vi "Color_Min_Max_ISOSPI.vi"(9 "datain":dbl[][](array[numeric]), 10 "valeur invalide":dbl, 11 "Table en entrée":refnum<vi>) -> ()   [LabVIEW 2020]
uses:
  <vilib>/Utility/miscctls.llb/LVRowAndColumnTypeDef.ctl
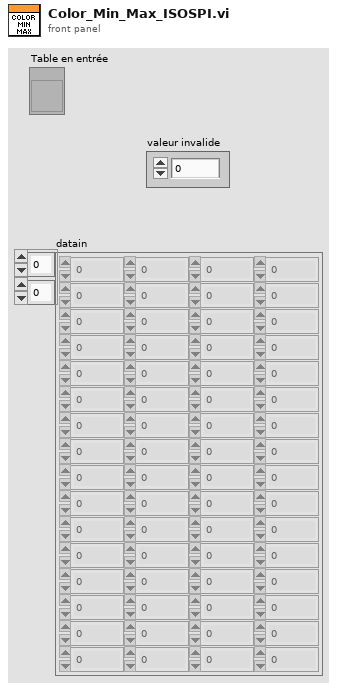
[diagram p1: front panel]
types:
  T1 = typedef "LVRowAndColumnTypeDef.ctl" = cluster{"Row":i32, "Column":i32}
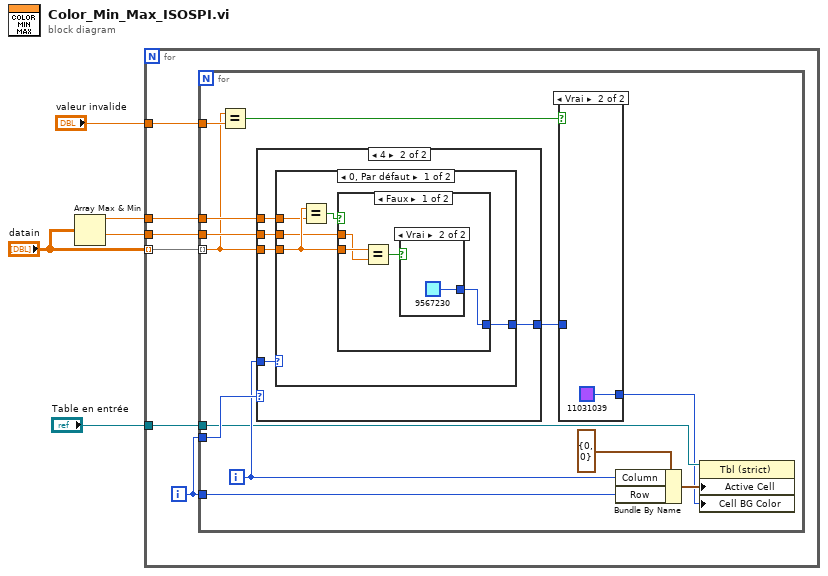
[diagram p0: block diagram]
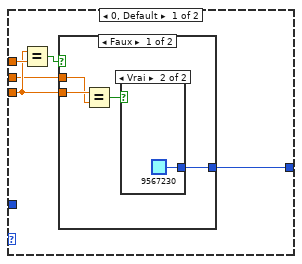
[diagram p3: hidden frame]
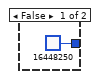
[diagram p4: hidden frame]
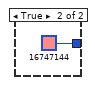
[diagram p5: hidden frame]
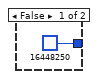
[diagram p6: hidden frame]
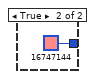
[diagram p7: hidden frame]
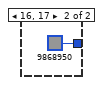
[diagram p8: hidden frame]
diagram:
  n1 = Array Max & Min ("Max. et min. d'un tableau")(array="datain") -> (max value=w3:dbl, min value=w2:dbl)  [unwired: 2 out]
  n2 = for {
    tunnel: "datain" -> [w11] mode=indexing
    tunnel: w3 -> [w9]
    tunnel: w2 -> [w8]
    tunnel: "Table en entrée" -> [w7]
    tunnel: "valeur invalide" -> [w6]
    i -> [w10]
    n3 = for {
      tunnel: w11 -> [w12] mode=indexing
      tunnel: w10 -> [w23]
      tunnel: w10 -> [w22]
      tunnel: w9 -> [w21]
      tunnel: w8 -> [w20]
      tunnel: w7 -> [w18]
      tunnel: w6 -> [w14]
      i -> [w19]
      n4 = Equal?(x=w12, y=w14) -> (x = y?=w13:bool)
      n5 = case shown="4" w22 {
        tunnel: w19 -> [_ w43]
        tunnel: w12 -> [w29 w41]
        tunnel: w21 -> [w31 w40]
        tunnel: w20 -> [w28 w39]
        tunnel: [w27 w42] -> w16
        frame 0, Default {
          n6 = Equal?(x=w29, y=w31) -> (x = y?=w30:bool)
          n7 = case shown="Faux" w30 {
            tunnel: w29 -> [w35 _]
            tunnel: w28 -> [w34 _]
            tunnel: [w32 u32 16747144] -> w27
            frame False {
              n8 = Equal?(x=w35, y=w34) -> (x = y?=w33:bool)
              n9 = case shown="Vrai" w33 {
                tunnel: [u32 16448250 u32 9567230] -> w32
                frame False {
                }
                frame True {
                }
              }
            }
            frame True {
            }
          }
        }
        frame 4 {
          n10 = case shown="0, Par défaut" w43 {
            tunnel: [w48 u32 9868950] -> w42
            tunnel: w41 -> [w47 _]
            tunnel: w40 -> [w46 _]
            tunnel: w39 -> [w44 _]
            frame 0, Default {
              n11 = Equal?(x=w47, y=w46) -> (x = y?=w45:bool)
              n12 = case shown="Faux" w45 {
                tunnel: w47 -> [w52 _]
                tunnel: w44 -> [w51 _]
                tunnel: [w49 u32 16747144] -> w48
                frame False {
                  n13 = Equal?(x=w52, y=w51) -> (x = y?=w50:bool)
                  n14 = case shown="Vrai" w50 {
                    tunnel: [u32 16448250 u32 9567230] -> w49
                    frame False {
                    }
                    frame True {
                    }
                  }
                }
                frame True {
                }
              }
            }
            frame 16, 17 {
            }
          }
        }
      }
      n15 = case shown="Vrai" w13 {
        tunnel: [w25 u32 11031039] -> w15
        tunnel: w16 -> [w25 _]
        frame False {
        }
        frame True {
        }
      }
      n16 = Bundle By Name(cluster=T1 {"Row"=0, "Column"=0} ("Cellule active:Cellule active"), "Column"=w19, "Row"=w23) -> (w17:T1)
      n17 = property class="Tbl (strict)"(reference=w18, "Active Cell"=w17, "Cell BG Color"=w15) -> ()  [unwired: 1 in, 2 out]
    }
  }
